vi "Recolor Front Panel.vi"(7 "QD Launch VI Panel?":bool, 8 "Error In":errorcluster, 11 "reference":refnum<vi>) -> (0 "Error Out":errorcluster, 1 "Changed?":bool, 3 "reference out":refnum<vi>)   [LabVIEW 2017]
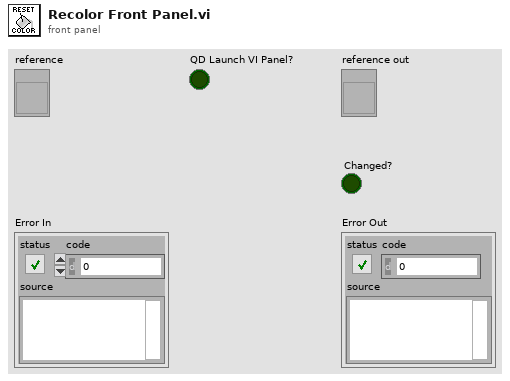
[diagram p1: front panel]
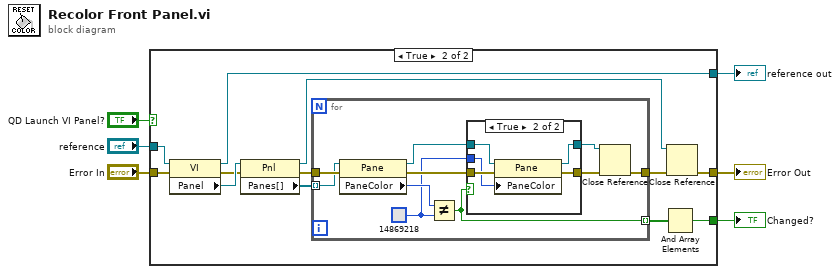
[diagram p0: block diagram]
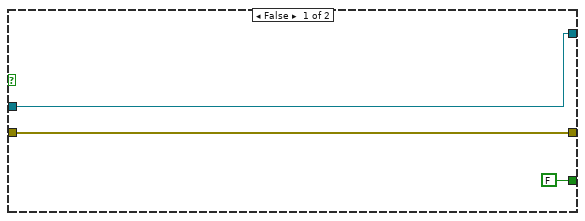
[diagram p2: hidden frame]
diagram:
  n1 = case shown="True" "QD Launch VI Panel?" {
    tunnel: "reference" -> [w9 w21]
    tunnel: [w8 w15] -> w5
    tunnel: "Error In" -> [w8 w13]
    tunnel: [FALSE w11] -> w3
    tunnel: [w9 w10] -> w2
    frame False {
    }
    frame True {
      n2 = property class="VI"(reference=w21, error in=w13) -> (reference out=w10:refnum<vi>, error out=w14:errorcluster, "Panel"=w20:refnum<vi>)
      n3 = property class="Pnl"(reference=w20, error in=w14) -> (reference out=w17:refnum<vi>, error out=w18:errorcluster, "Panes[]"=w19:refnum<vi>[])
      n4 = for {
        tunnel: w19 -> [w30] mode=indexing
        tunnel: w18 -> [w31]
        tunnel: [w22] -> w16
        tunnel: [w25] -> w12 mode=indexing
        w26 = u32 14869218
        n5 = property class="Pane"(reference=w30, error in=w31) -> (reference out=w29:refnum<vi>, error out=w28:errorcluster, "PaneColor"=w27:u32)
        n6 = Not Equal?(x=w27, y=w26) -> (x != y?=w25:bool)
        n7 = case shown="True" w25 {
          tunnel: w29 -> [w33 w38]
          tunnel: w28 -> [w32 w37]
          tunnel: w26 -> [_ w36]
          tunnel: [w32 w35] -> w24
          tunnel: [w33 w34] -> w23
          frame False {
          }
          frame True {
            n8 = property class="Pane"(reference=w38, error in=w37, "PaneColor"=w36) -> (reference out=w34:refnum<vi>, error out=w35:errorcluster)
          }
        }
        n9 = Close Reference(reference=w23, error in (no error)=w24) -> (error out=w22:errorcluster)
      }
      n10 = And Array Elements(Boolean array=w12) -> (logical AND=w11:bool)
      n11 = Close Reference(reference=w17, error in (no error)=w16) -> (error out=w15:errorcluster)
    }
  }
  "Error Out" <- w5
  "Changed?" <- w3
  "reference out" <- w2
